vi "Read Interlocks.vi"(8 "error in (no error)":errorcluster, 9 "Write if not found? (T)":bool=TRUE, 10 "Variable Names":string[](array[string]), 11 "Interlocks (.ini)":path) -> (0 "error out":errorcluster, 1 "Modified?":bool, 2 "Variable Interlocks":string[](array[string]))   [LabVIEW 2022 SP3, in "Interlocks.lvlib"]
uses:
  Interlocks.lvlib
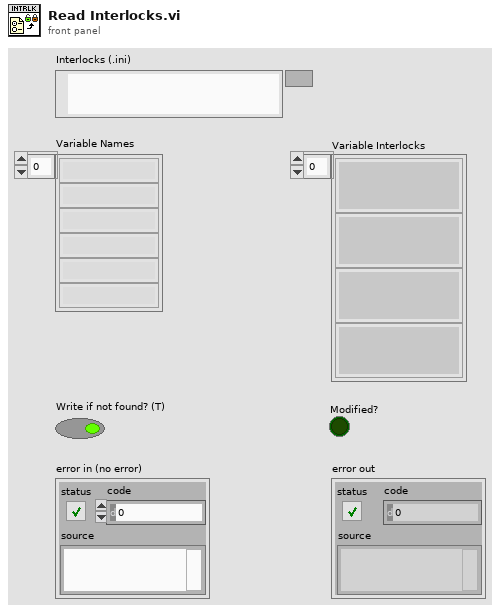
[diagram p1: front panel]
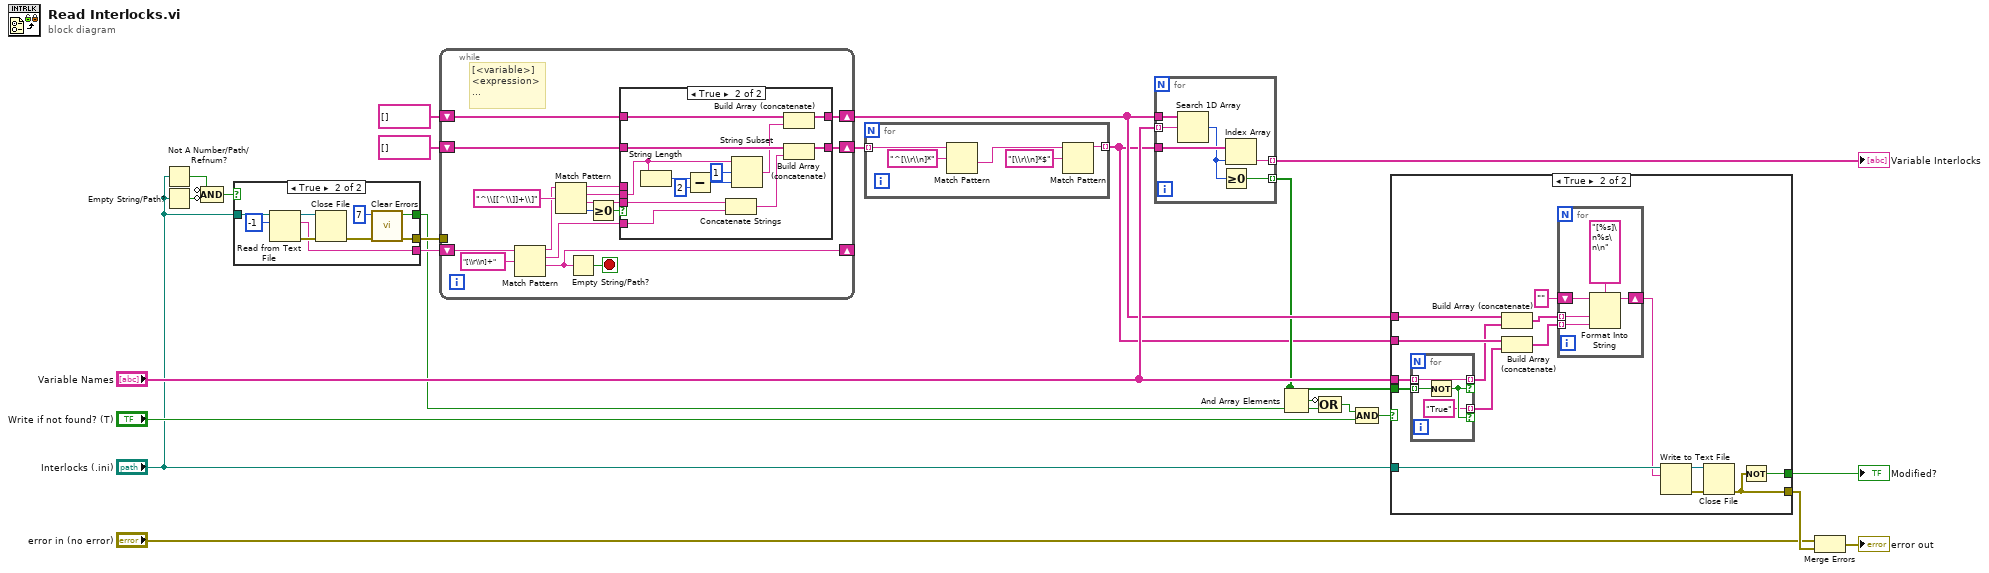
[diagram p0: block diagram]
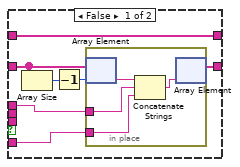
[diagram p3: hidden frame]
diagram:
  n1 = Not A Number/Path/Refnum?(number/path/refnum="Interlocks (.ini)") -> (NaN/Path/Refnum?=w8:bool)
  n2 = Empty String/Path?(string/path="Interlocks (.ini)") -> (empty?=w7:bool)
  n3 = Compound Arithmetic op=AND(invert w8, invert w7) -> (w6:bool)
  n4 = case shown="True" w6 {
    tunnel: [_ w29] -> w19
    tunnel: [_ w27] -> w13
    tunnel: "Interlocks (.ini)" -> [_ w25]
    tunnel: [_ w24] -> w9
    frame False {
    }
    frame True {
      n5 = Read from Text File(file (use dialog)=w25, count=-1) -> (refnum out=w31:refnum<file>, text=w29:string, error out=w32:errorcluster)  [unwired: 2 in, 1 out]
      n6 = Close File(refnum=w31, error in=w32) -> (error out=w28:errorcluster)  [unwired: 1 out]
      n7 = call <vilib>:"Clear Errors.vi"("error in (no error)"=w28, "specific error code to clear (0: all)"=7) -> ("error out"=w27:errorcluster, "specific error cleared?"=w24:bool)  [unwired: 4 in]
    }
  }
  n8 = while {
    shift-right: [w44] -> _
    shift-left: w19 -> [w46]
    shift-right: [w40] -> w2
    shift-left: string[] [] -> [w39]
    shift-right: [w37] -> w15
    shift-left: string[] [] -> [w38]
    tunnel: w13 -> [_]
    stop <- w43 stop-if-true
    # "[<variable>]\n<expression>\n..."
    n9 = Match Pattern(string=w46, regular expression="[\\r\\n]+") -> (before substring=w45:string, match substring=w34:string, after substring=w44:string)  [unwired: 1 in, 1 out]
    n10 = Match Pattern(string=w45, regular expression="^\\[[^\\]]+\\]") -> (before substring=w36:string, match substring=w33:string, after substring=w35:string, offset past match=w42:i32)  [unwired: 1 in]
    n11 = Empty String/Path?(string/path=w44) -> (empty?=w43:bool)
    n12 = Greater Or Equal To 0?(x=w42) -> (x >= 0?=w41:bool)
    n13 = case shown="True" w41 {
      tunnel: [w50 w70] -> w40
      tunnel: w39 -> [w54 w72]
      tunnel: w38 -> [w55 w71]
      tunnel: [w55 w69] -> w37
      tunnel: w36 -> [w49 _]
      tunnel: w35 -> [_ w68]
      tunnel: w34 -> [w51 w66]
      tunnel: w33 -> [_ w64]
      frame False {
        n14 = Array Size(array=w54) -> (size(s)=w53:i32)
        n15 = Decrement(x=w53) -> (x-1=w52:i32)
        n16 = in-place {
          in-place-border: w49 -> [w58]
          in-place-border: w51 -> [w57]
          n17 = in-place-array #1(w54, w52) -> (w59:string)
          n18 = Concatenate Strings(w59, w58, w57) -> (w56:string)
          n19 = in-place-array #1(w56) -> (w50:string[])  [unwired: 1 out]
        }
      }
      frame True {
        n20 = String Length(string=w64) -> (length=w63:i32)
        n21 = Subtract(x=w63, y=2 ("offset (0)")) -> (x-y=w62:i32)
        n22 = Concatenate Strings(w68, w66) -> (w67:string)
        n23 = String Subset(string=w64, offset (0)=1, length (rest)=w62) -> (substring=w60:string)
        n24 = Build Array (concatenate)(w71, w60) -> (w69:string[])
        n25 = Build Array (concatenate)(w72, w67) -> (w70:string[])
      }
    }
  }
  n26 = for {
    tunnel: w2 -> [w74] mode=indexing
    tunnel: [w76] -> w1 mode=indexing
    n27 = Match Pattern(string=w74, regular expression="^[\\r\\n]*") -> (after substring=w73:string)  [unwired: 1 in, 3 out]
    n28 = Match Pattern(string=w73, regular expression="[\\r\\n]*$") -> (before substring=w76:string)  [unwired: 1 in, 3 out]
  }
  n29 = for {
    tunnel: w15 -> [w83]
    tunnel: "Variable Names" -> [w82] mode=indexing
    tunnel: w1 -> [w81]
    tunnel: [w80] -> w23 mode=indexing
    tunnel: [w78] -> w14 mode=indexing
    n30 = Search 1D Array(1D array=w83, element=w82) -> (index of element=w79:i32)  [unwired: 1 in]
    n31 = Greater Or Equal To 0?(x=w79) -> (x >= 0?=w78:bool)
    n32 = Index Array(array=w81, index=w79) -> (element=w80:string)
  }
  "Variable Interlocks" <- w23
  n33 = And Array Elements(Boolean array=w14) -> (logical AND=w11:bool)
  n34 = Compound Arithmetic op=OR(invert w11, w9) -> (w10:bool)
  n35 = Compound Arithmetic op=AND(w10, "Write if not found? (T)") -> (w16:bool)
  n36 = case shown="True" w16 {
    tunnel: "Interlocks (.ini)" -> [_ w97]
    tunnel: [_ w85] -> w22
    tunnel: w15 -> [_ w95]
    tunnel: w1 -> [_ w94]
    tunnel: "Variable Names" -> [_ w89]
    tunnel: w14 -> [_ w88]
    tunnel: [_ w84] -> w3
    frame False {
    }
    frame True {
      n37 = for {
        tunnel: w89 -> [w102] mode=indexing
        tunnel: w88 -> [w101] mode=indexing
        tunnel: [w102] -> w87 mode=indexing if=w100
        tunnel: ["True"] -> w86 mode=indexing if=w100
        n38 = Not(x=w101) -> (.not. x?=w100:bool)
      }
      n39 = Build Array (concatenate)(w95, w87) -> (w90:string[])
      n40 = Build Array (concatenate)(w94, w86) -> (w91:string[])
      n41 = for {
        tunnel: w90 -> [w106] mode=indexing
        tunnel: w91 -> [w107] mode=indexing
        shift-right: [w105] -> w92
        shift-left: "" -> [w104]
        n42 = Format Into String(format string="[%s]\n%s\n\n", initial string=w104, w106, w107) -> (resulting string=w105:string)  [unwired: 1 in, 1 out]
      }
      n43 = Write to Text File(file (use dialog)=w97, text=w92) -> (refnum out=w96:refnum<file>, error out=w98:errorcluster)  [unwired: 2 in, 1 out]
      n44 = Close File(refnum=w96, error in=w98) -> (error out=w85:errorcluster)  [unwired: 1 out]
      n45 = Not(x=w85) -> (.not. x?=w84:bool)
    }
  }
  "Modified?" <- w3
  n46 = Merge Errors("error in (no error)", w22) -> (→"error out":errorcluster)
